vi "Configure Timebase.vi"   [LabVIEW 2023, in "Keysight-DSQx3014T.lvlib"]
doc: "Configures timebase settings."
uses:
  Keysight-DSQx3014T.lvlib
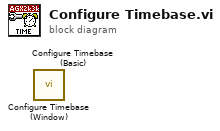
[diagram p0: block diagram]
diagram:
  n1 = call "Configure Timebase (Window).vi"() -> ()  [unwired: 14 in, 2 out]
  n2 = call "Configure Timebase (Basic).vi"() -> ()  [unwired: 14 in, 2 out]
